vi "StopDI.vi"(8 "error in (no error)":errorcluster, 10 "gRPCid":T5, 11 "DIOSessions In":T1={"Array of DI Sessions"=[], "Array of DO Sessions"=[], "Stream ReadDI"={"gRPCid ReadDI"=0, "DISessionName"="", "Stream Status ReadDI"=FALSE, "Async Stop ReadDI Queue"=refnum, "DI Task"="", "ms to wait"=500}}) -> (0 "error out":errorcluster, 3 "DIOSessions Out":T1={"Array of DI Sessions"=[], "Array of DO Sessions"=[], "Stream ReadDI"={"gRPCid ReadDI"=0, "DISessionName"="", "Stream Status ReadDI"=FALSE, "Async Stop ReadDI Queue"=refnum, "DI Task"="", "ms to wait"=500}})   [LabVIEW 2019, in "ctet_dio_User Library.lvlib"]
uses:
  ctet_dio_User Library.lvlib
  Servers/ctet_dio/gRPC lvSupport/Server API/typeDefs/grpcId.ctl
  Types/DIOSessions.ctl
  Types/DISession.ctl
  Types/DOSession.ctl
  Types/StreamReadDI.ctl
  Servers/ctet_dio/ctet_dio Class/RPC Messages/measurementservice_StopDIResponse/measurementservice_StopDIResponse_Data.ctl
  Servers/ctet_dio/ctet_dio Class/RPC Messages/measurementservice_ErrorOut/measurementservice_ErrorOut_Data.ctl
  Servers/ctet_dio/ctet_dio Class/ctet_dio.lvclass
  Servers/ctet_dio/gRPC lvSupport/gprc-lvsupport.lvlib
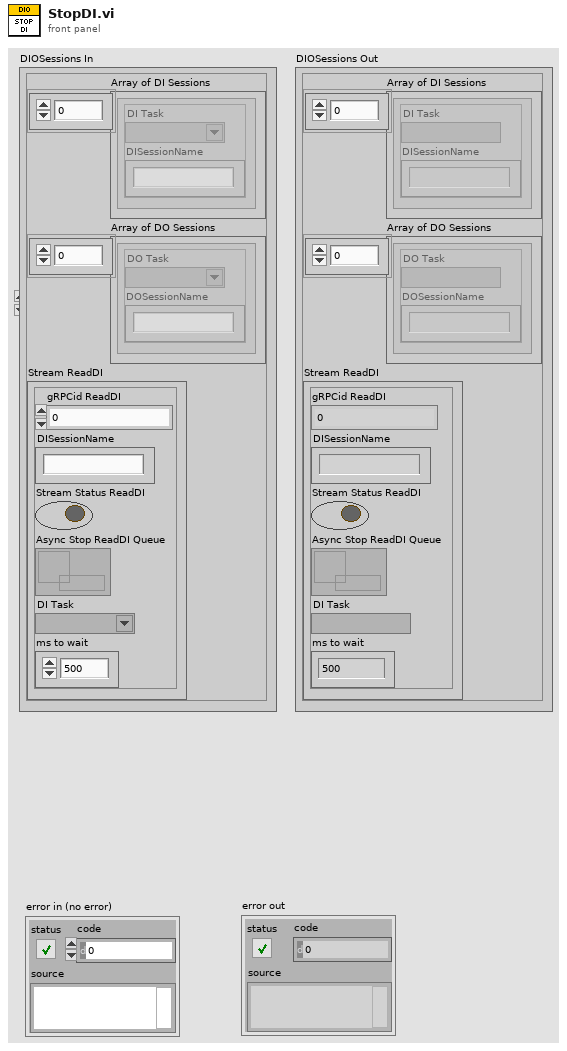
[diagram p1: front panel]
types:
  T1 = typedef "ctet_dio_User Library.lvlib/DIOSessions.ctl" = cluster{"Array of DI Sessions":T2[], "Array of DO Sessions":T3[], "Stream ReadDI":T4}
  T2 = typedef "ctet_dio_User Library.lvlib/DISession.ctl" = cluster{"DI Task":refnum<k21>, "DISessionName":string}
  T3 = typedef "ctet_dio_User Library.lvlib/DOSession.ctl" = cluster{"DO Task":refnum<k21>, "DOSessionName":string}
  T4 = typedef "ctet_dio_User Library.lvlib/StreamReadDI.ctl" = cluster{"gRPCid ReadDI":T5, "DISessionName":string, "Stream Status ReadDI":bool, "Async Stop ReadDI Queue":refnum<queue>, "DI Task":refnum<k21>, "ms to wait":u32}
  T5 = typedef "ctet_dio.lvlib/gprc-lvsupport.lvlib/grpcId.ctl" = u64
  T6 = typedef "ctet_dio.lvlib/ctet_dio.lvclass/measurementservice_ErrorOut_Data.ctl" = cluster{"errCode":i64, "errMessage":string}
  T7 = typedef "ctet_dio.lvlib/ctet_dio.lvclass/measurementservice_StopDIResponse_Data.ctl" = cluster{"DISessionName":string, "error":T6}
  T8 = typedef "ctet_dio.lvlib/ctet_dio.lvclass/measurementservice_StopDIRequest_Data.ctl" = cluster{"DISessionName":string}
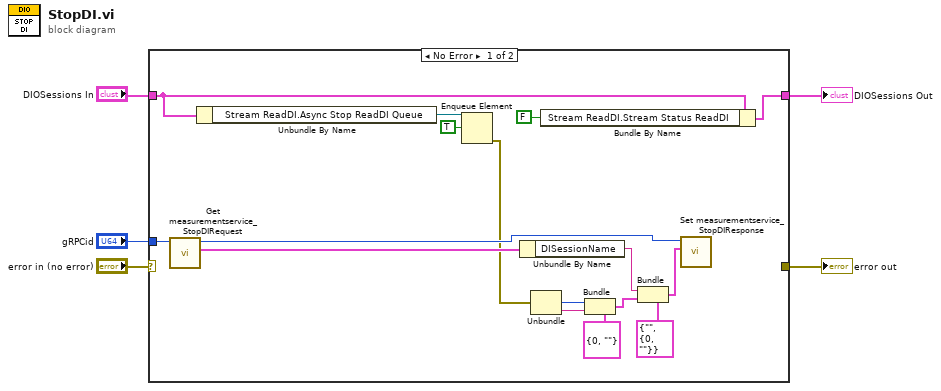
[diagram p0: block diagram]
diagram:
  n1 = case shown="No Error" "error in (no error)" {
    selector: "error in (no error)" -> [_ w23]
    tunnel: [_ w23] -> w5
    tunnel: "gRPCid" -> [w21 _]
    tunnel: "DIOSessions In" -> [w17 w22]
    tunnel: [w16 w22] -> w1
    frame No Error {
      n2 = call "Get measurementservice_StopDIRequest.vi"("gRPCid"=w21) -> ("Message Data"=w13:T8, "gRPCid out"=w7:T5)  [unwired: 8 in, 1 out]
      n3 = Unbundle By Name(w17) -> ("Stream ReadDI.Async Stop ReadDI Queue"=w20:refnum<queue>)
      n4 = Enqueue Element(queue=w20, element=TRUE) -> (error out=w6:errorcluster)  [unwired: 2 in, 2 out]
      n5 = Unbundle By Name(w13) -> ("DISessionName"=w12:string)
      n6 = Unbundle(w6) -> ("code"=w9:i32, "source"=w8:string)  [unwired: 1 out]
      n7 = Bundle By Name(cluster=w17, "Stream ReadDI.Stream Status ReadDI"=FALSE) -> (w16:T1)
      n8 = Bundle(cluster=T6 {"errCode"=0, "errMessage"=""} ("error"), "errCode"=w9, "errMessage"=w8) -> (w10:T6)
      n9 = Bundle(cluster=T7 {"DISessionName"="", "error"={"errCode"=0, "errMessage"=""}} ("measurementservice_StopDIResponse_Data"), "DISessionName"=w12, "error"=w10) -> (w14:T7)
      n10 = call "Set measurementservice_StopDIResponse.vi"("Message Data"=w14, "gRPCid"=w7) -> ()  [unwired: 9 in, 1 out]
    }
    frame Error {
    }
  }
  "error out" <- w5
  "DIOSessions Out" <- w1
